vi "Set (Boolean Array Data Type).vi"(5 "Tag":string, 7 "error in (no error)":errorcluster, 9 "Value":bool[](array[boolean]), 10 "ByRef Variant Repsitory in":refnum<data-value>) -> (0 "error out":errorcluster)   [LabVIEW 2015, in "ByRef Variant Repository.lvlib"]
uses:
  ByRef Variant Repository.lvlib
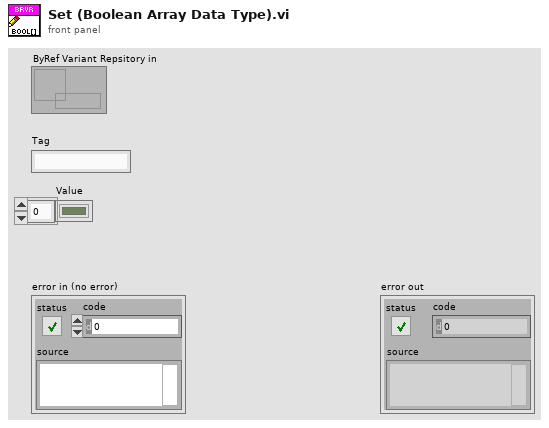
[diagram p1: front panel]
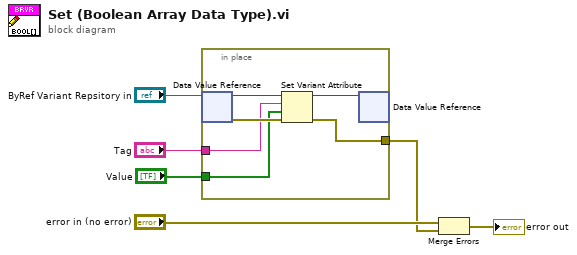
[diagram p0: block diagram]
diagram:
  n1 = in-place {
    in-place-border: [w9] -> w4
    in-place-border: "Tag" -> [w8]
    in-place-border: "Value" -> [w7]
    n2 = in-place-dvr #1("ByRef Variant Repsitory in") -> (w11:variant, w12:errorcluster)
    n3 = Set Variant Attribute(Variant=w11, name=w8, value=w7, error in=w12) -> (Variant out=w10:variant, error out=w9:errorcluster)  [unwired: 1 out]
    n4 = in-place-dvr #1(w10) -> ()  [unwired: 2 out]
  }
  n5 = Merge Errors("error in (no error)", w4) -> (→"error out":errorcluster)
